vi "Write Label at Path(String).vi"(8 "error in (no error)":errorcluster, 9 "Name":string, 10 "Path String":string, 11 "Variant in":variant) -> (0 "error out":errorcluster, 3 "Variant out":variant)   [LabVIEW 2017, in "Variant Data Manipulation.lvlib"]
uses:
  Variant Data Manipulation.lvlib
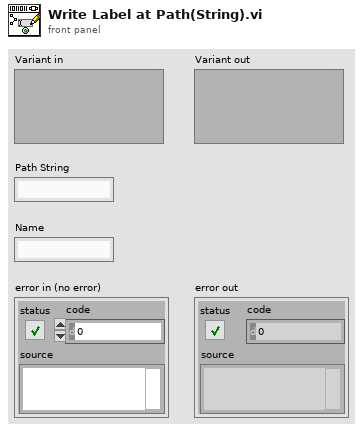
[diagram p1: front panel]
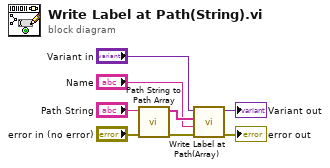
[diagram p0: block diagram]
diagram:
  n1 = call "Path String to Path Array.vi"("error in (no error)"="error in (no error)", "Path String"="Path String") -> ("error out"=w8:errorcluster, "Path Array"=w7:string[])  [unwired: 8 in]
  n2 = call "Write Label at Path(Array).vi"("error in (no error)"=w8, "Name"="Name", "Path in"=w7, "Variant in"="Variant in") -> ("error out"=→"error out":errorcluster, "Variant out"=→"Variant out":variant)  [unwired: 6 in]
